vi "Manage.vi"(8 "error in":errorcluster, 10 "ToDo":T2, 11 "Database IN":T1[](array[typedef]) {"Balance" format="%#.2f"; "Account Number" format="%_1f"}) -> (0 "error out":errorcluster, 3 "Database OUT":T1[](array[typedef]) {"Balance" format="%#.2f"; "Account Number" format="%_1f"})   [LabVIEW 2020]
doc: "Manage database by open / update an account"
uses:
  Controls/Todo.ctl
  Controls/Account Database.ctl
  <vilib>/Utility/xml.llb/Read From XML File(string).vi
  <vilib>/Utility/xml.llb/Write to XML File(string).vi
panel:
  # "[Covers: CD1A]"
  # "[Covers: CD1B]"
  # "[Covers: CD1C]"
  # "[Covers: CD1D]"
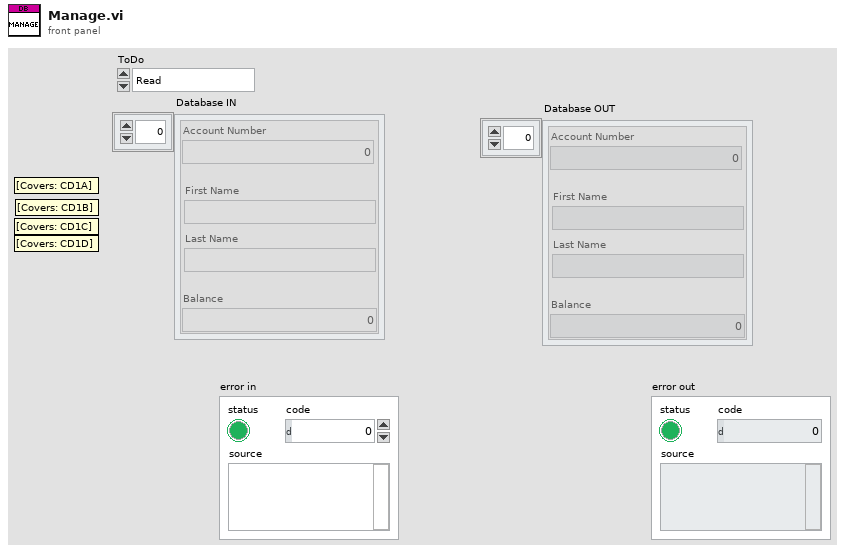
[diagram p1: front panel]
types:
  T1 = typedef "Account Database.ctl" = cluster{"Account Number":i32, "First Name":string, "Last Name":string, "Balance":dbl}
  T2 = typedef "Todo.ctl" = enum16{"Read", "Update"}
  T3 = enum16{"open", "replace", "create", "open or create", "replace or create", "replace or create with confirmation"}
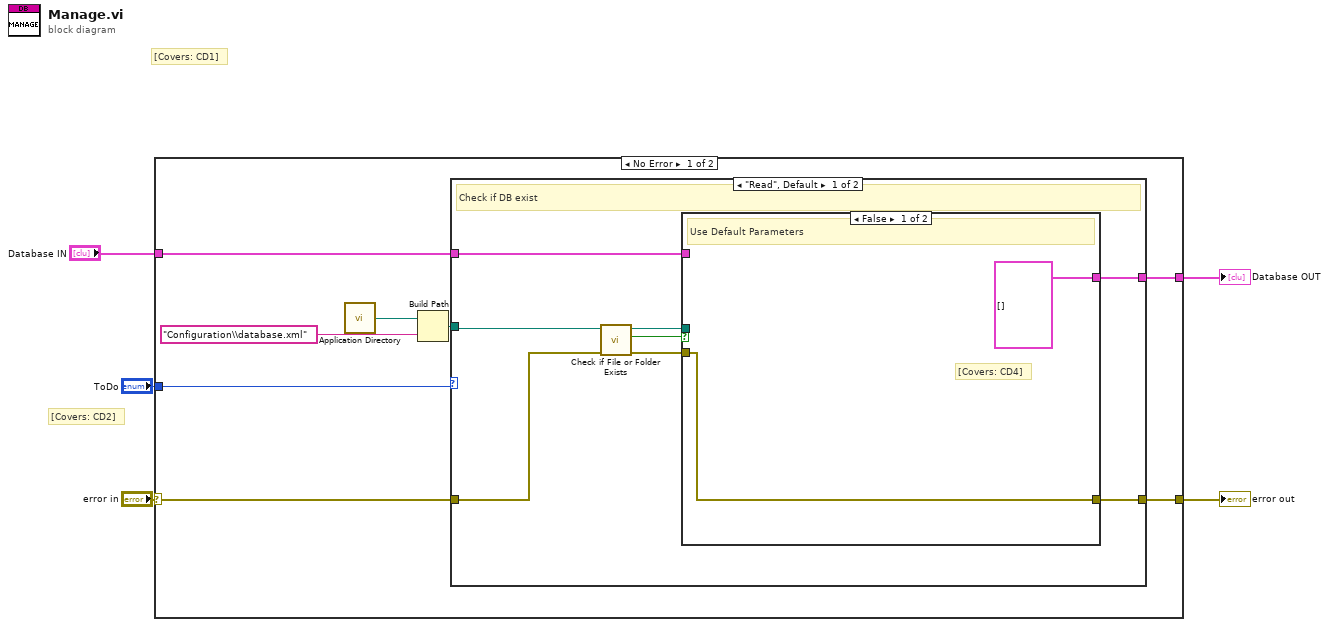
[diagram p0: block diagram]
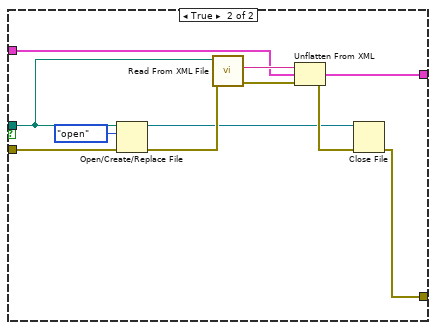
[diagram p2: hidden frame]
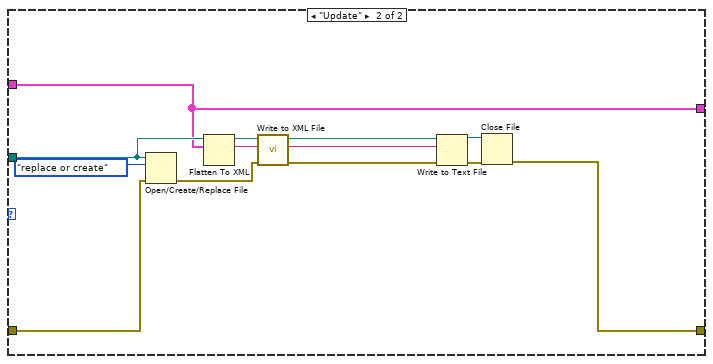
[diagram p3: hidden frame]
diagram:
  # "[Covers: CD2]"
  # "[Covers: CD1]"
  n1 = case shown="No Error" "error in" {
    selector: "error in" -> [w9 w48]
    tunnel: [w6 w48] -> w4
    tunnel: "ToDo" -> [w13 _]
    tunnel: "Database IN" -> [w8 w47]
    tunnel: [w7 w47] -> w1
    frame No Error {
      n2 = call <vilib>:"Application Directory.vi"() -> ("Application Directory"=w12:path)
      n3 = Build Path(base path=w12, name or relative path="Configuration\\database.xml" ("string")) -> (appended path=w10:path)
      n4 = case shown="\"Read\", Default" w13 {
        tunnel: w10 -> [w20 w43]
        tunnel: w9 -> [w21 w45]
        tunnel: w8 -> [w15 w41]
        tunnel: [w17 w41] -> w7
        tunnel: [w14 w44] -> w6
        frame "Read", Default {
          # "Check if DB exist"
          n5 = call <vilib>:"Check if File or Folder Exists.vi"("error in (no error)"=w21, "path"=w20) -> ("error out"=w18:errorcluster, "file or folder exists?"=w19:bool, "dup path"=w16:path)  [unwired: 7 in]
          n6 = case shown="False" w19 {
            tunnel: w18 -> [w22 w34]
            tunnel: [T1[] [] ("Database") w27] -> w17
            tunnel: w16 -> [_ w32]
            tunnel: w15 -> [_ w28]
            tunnel: [w22 w24] -> w14
            frame False {
              # "[Covers: CD4]"
              # "Use Default Parameters"
            }
            frame True {
              n7 = Open/Create/Replace File(file path (use dialog)=w32, error in=w34, operation (0:open)=T3."open") -> (refnum out=w25:refnum<file>, error out=w31:errorcluster)  [unwired: 3 in, 1 out]
              n8 = call-poly <vilib>:"Read From XML File.vi"("error in (no error)"=w31, "XML File Path"=w32) -> ("error out"=w29:errorcluster, "XML Elements"=w30:string)  [unwired: 7 in, 1 out]
              n9 = Unflatten From XML(xml string=w30, type=w28, error in (no error)=w29) -> (value=w27:T1[], error out=w26:errorcluster)
              n10 = Close File(refnum=w25, error in=w26) -> (error out=w24:errorcluster)  [unwired: 1 out]
            }
          }
        }
        frame "Update" {
          n11 = Open/Create/Replace File(file path (use dialog)=w43, error in=w45, operation (0:open)=T3."replace or create") -> (error out=w42:errorcluster)  [unwired: 3 in, 2 out]
          n12 = Flatten To XML(6:w41) -> (2:w40:string)
          n13 = call-poly <vilib>:"Write to XML File.vi"("error in (no error)"=w42, "XML Input"=w40, "XML File Path"=w43) -> ("error out"=w39:errorcluster, "XML String"=w37:string, "XML File Path(duplicate)"=w38:path)  [unwired: 6 in]
          n14 = Write to Text File(file (use dialog)=w38, text=w37, error in=w39) -> (refnum out=w35:refnum<file>, error out=w36:errorcluster)  [unwired: 1 in, 1 out]
          n15 = Close File(refnum=w35, error in=w36) -> (error out=w44:errorcluster)  [unwired: 1 out]
        }
      }
    }
    frame Error {
    }
  }
  "error out" <- w4
  "Database OUT" <- w1
